vi "Configure Frequency Domain Measurement.vi"(0 "VISA resource name":refnum<visa-resource-name>, 1 "Number of Adjacent Channels (1)":i8=1 min=1 max=3 step=1, 2 "Percentage of Power (60%)":dbl=60.0 min=60.0 max=99.9 step=0.1 format="%#_g %", 5 "Measurement (0:None)":u16(ring) items=["None", "Channel Power", "Adjacent Channel Power Ratio", "Occupied Bandwidth"], 7 "Channel BandWidth (0)":dbl, 9 "Units (0:Hz)":u16(ring) items=["Hz", "KHz", "MHz", "GHz"], 11 "error in (no error)":errorcluster, 12 "Channel Spacing (14 Hz)":dbl=14.0 min=14.0, 13 "Spacing Units (0:Hz)":u16(ring) items=["Hz", "kHz", "MHz", "GHz"]) -> (4 "VISA resource name out":refnum<visa-resource-name>, 15 "error out":errorcluster)   [LabVIEW 2017, in "Scope.lvlib" / "Tektronix DPO MSO 2000 4000 Series.lvlib"]
doc: "Configures the Frequency Domain Measurements and their parameters for the MDO series oscilloscopes.\n\n<B>Note:</B>\n This VI is applicable only to <B>MDO series</B> oscilloscopes."
uses:
  Tektronix DPO MSO 2000 4000 Series.lvlib
panel:
  # "All Measurements"
  # "Adjacent Channel Power Ratio Measurement"
  # "Occupied Bandwidth Measurement"
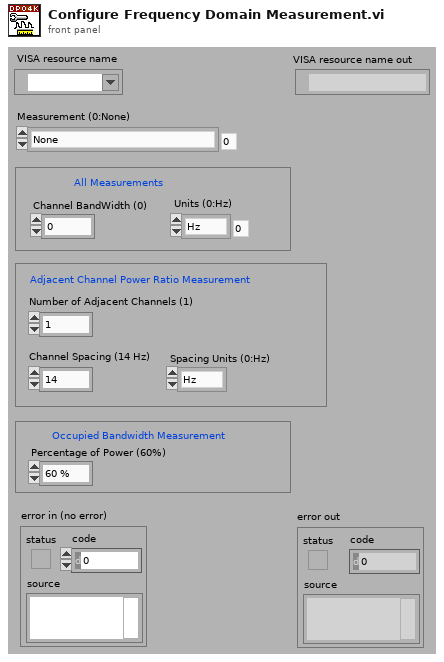
[diagram p1: front panel]
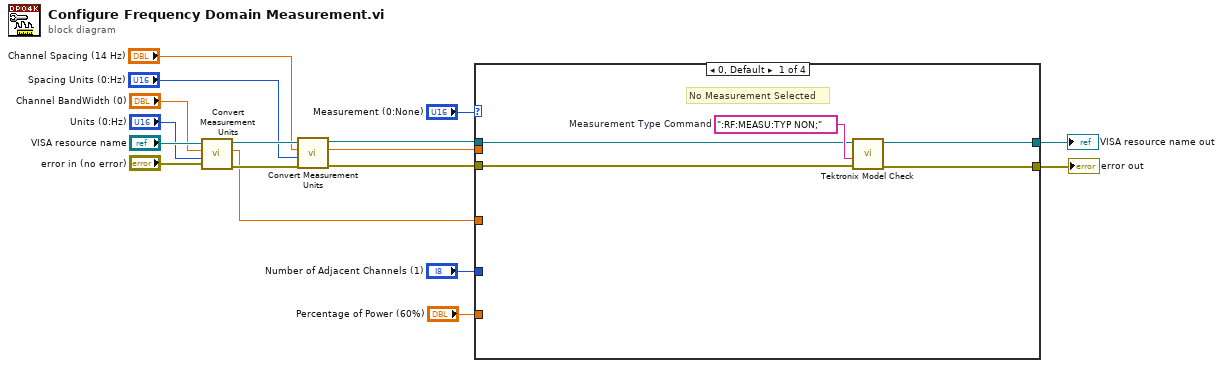
[diagram p0: block diagram]
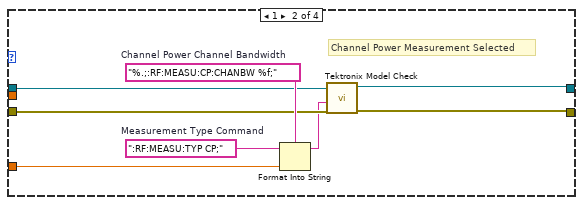
[diagram p2: hidden frame]
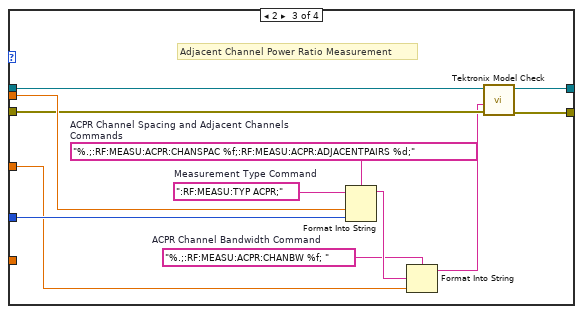
[diagram p3: hidden frame]
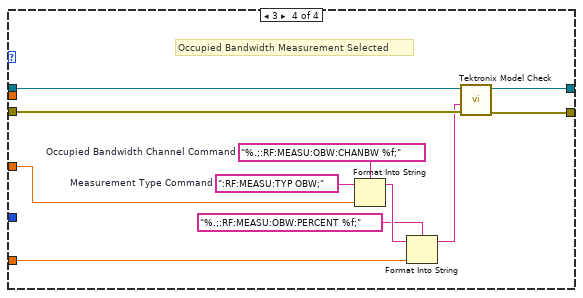
[diagram p4: hidden frame]
diagram:
  n1 = call "Convert Measurement Units.vi"("error in (no error)"="error in (no error)", "Units (0:Hz)"="Units (0:Hz)", "Measurement Value (0)"="Channel BandWidth (0)", "VISA resource name"="VISA resource name") -> ("error out"=w8:errorcluster, "Final Value"=w3:dbl, "VISA resource name out"=w7:refnum<visa-resource-name>)  [unwired: 5 in]
  n2 = call "Convert Measurement Units.vi"("error in (no error)"=w8, "Units (0:Hz)"="Spacing Units (0:Hz)", "Measurement Value (0)"="Channel Spacing (14 Hz)", "VISA resource name"=w7) -> ("error out"=w1:errorcluster, "Final Value"=w2:dbl, "VISA resource name out"=w4:refnum<visa-resource-name>)  [unwired: 5 in]
  n3 = case shown="0, Default" "Measurement (0:None)" {
    tunnel: w4 -> [w21 w27 w35 w47]
    tunnel: [w20 w24 w32 w44] -> w16
    tunnel: [w19 w23 w31 w43] -> w15
    tunnel: "Number of Adjacent Channels (1)" -> [_ _ w40 _]
    tunnel: "Percentage of Power (60%)" -> [_ _ _ w48]
    tunnel: w3 -> [_ w29 w36 w51]
    tunnel: w2 -> [_ _ w39 _]
    tunnel: w1 -> [w18 w26 w34 w46]
    frame 0, Default {
      w22 = ":RF:MEASU:TYP NON;"  # Measurement Type Command
      # "No Measurement Selected"
      n4 = call "Tektronix Model Check.vi"("error in (no error)"=w18, "Command String"=w22, "VISA resource name"=w21) -> ("error out"=w19:errorcluster, "VISA resource name out"=w20:refnum<visa-resource-name>)  [unwired: 7 in]
    }
    frame 1 {
      w30 = "%.;:RF:MEASU:CP:CHANBW %f;"  # Channel Power Channel Bandwidth
      w28 = ":RF:MEASU:TYP CP;"  # Measurement Type Command
      # "Channel Power Measurement Selected"
      n5 = Format Into String(format string=w30, initial string=w28, w29) -> (resulting string=w25:string)  [unwired: 1 in, 1 out]
      n6 = call "Tektronix Model Check.vi"("error in (no error)"=w26, "Command String"=w25, "VISA resource name"=w27) -> ("error out"=w23:errorcluster, "VISA resource name out"=w24:refnum<visa-resource-name>)  [unwired: 7 in]
    }
    frame 2 {
      w37 = "%.;:RF:MEASU:ACPR:CHANBW %f; "  # ACPR Channel Bandwidth Command
      w42 = "%.;:RF:MEASU:ACPR:CHANSPAC %f;:RF:MEASU:ACPR:ADJACENTPAIRS %d;"  # ACPR Channel Spacing and Adjacent Channels Commands
      w41 = ":RF:MEASU:TYP ACPR;"  # Measurement Type Command
      # "Adjacent Channel Power Ratio Measurement"
      n7 = Format Into String(format string=w42, initial string=w41, w39, w40) -> (resulting string=w38:string)  [unwired: 1 in, 1 out]
      n8 = Format Into String(format string=w37, initial string=w38, w36) -> (resulting string=w33:string)  [unwired: 1 in, 1 out]
      n9 = call "Tektronix Model Check.vi"("error in (no error)"=w34, "Command String"=w33, "VISA resource name"=w35) -> ("error out"=w31:errorcluster, "VISA resource name out"=w32:refnum<visa-resource-name>)  [unwired: 7 in]
    }
    frame 3 {
      w52 = "%.;:RF:MEASU:OBW:CHANBW %f;"  # Occupied Bandwidth Channel Command
      w53 = ":RF:MEASU:TYP OBW;"  # Measurement Type Command
      # "Occupied Bandwidth Measurement Selected"
      n10 = Format Into String(format string=w52, initial string=w53, w51) -> (resulting string=w50:string)  [unwired: 1 in, 1 out]
      n11 = Format Into String(format string="%.;:RF:MEASU:OBW:PERCENT %f;", initial string=w50, w48) -> (resulting string=w45:string)  [unwired: 1 in, 1 out]
      n12 = call "Tektronix Model Check.vi"("error in (no error)"=w46, "Command String"=w45, "VISA resource name"=w47) -> ("error out"=w43:errorcluster, "VISA resource name out"=w44:refnum<visa-resource-name>)  [unwired: 7 in]
    }
  }
  "error out" <- w15
  "VISA resource name out" <- w16
